vi "Write ClkHandle.vi"(8 "error in (no error)":errorcluster, 10 "ClkHandle":variant, 11 "SensorBase in":refnum<class "SensorBase.lvclass">) -> (0 "error out":errorcluster, 3 "SensorBase out":refnum<class "SensorBase.lvclass">)   [LabVIEW 2018, in "SensorPlugins.lvlib" / "SensorBase.lvclass"]
uses:
  SensorBase.lvclass
  SensorBase.lvclass/SensorBase.ctl
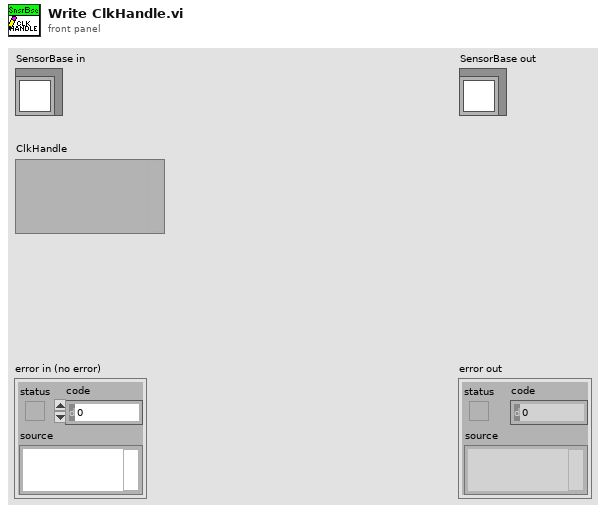
[diagram p1: front panel]
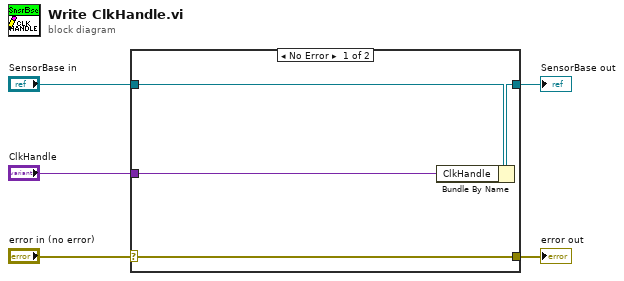
[diagram p0: block diagram]
diagram:
  n1 = case shown="No Error" "error in (no error)" {
    selector: "error in (no error)" -> [w9 w10]
    tunnel: [w9 w10] -> w4
    tunnel: [w7 w11] -> w2
    tunnel: "SensorBase in" -> [w8 w11]
    tunnel: "ClkHandle" -> [w6 _]
    frame No Error {
      n2 = Bundle By Name(cluster=w8, "ClkHandle"=w6) -> (w7:refnum<class "SensorBase.lvclass">)
    }
    frame Error {
    }
  }
  "error out" <- w4
  "SensorBase out" <- w2
